vi "load engine runtime.vi"(8 "error in":errorcluster, 10 "engine configuration in":T1, 11 "Target Runtime in":refnum<class "PL_Target Runtime.lvclass">) -> (0 "error out":errorcluster, 1 "Module Runtime Objects":refnum<class "TBM module execution interface.lvclass">[](array[class]), 2 "Engine Runtime Object":refnum<class "Engine Runtime Interface.lvclass">, 3 "Target Runtime out":refnum<class "PL_Target Runtime.lvclass">)   [LabVIEW 2013, in "PL_Target Runtime.lvclass"]
doc: "A helper function which takes a single engine configuration (1 engine configuration object and N module configuration objects) and loads the runtime objects associated with each configuration object."
uses:
  PL_Target Runtime.lvclass
  platypus configuration/engines cluster.ctl
  <vilib>/NI/Module Execution Interface/Engine Configuration/engine configuration.lvclass
  <vilib>/NI/Tag Bus Module Framework/module configuration/TBM module configuration.lvclass
  <vilib>/NI/Module Execution Interface/Engine Runtime/Engine Runtime Interface.lvclass
  <vilib>/NI/Tag Bus Module Framework/runtime/TBM module execution interface.lvclass
  platypus configuration/PLConfigurationSerializer.lvlib
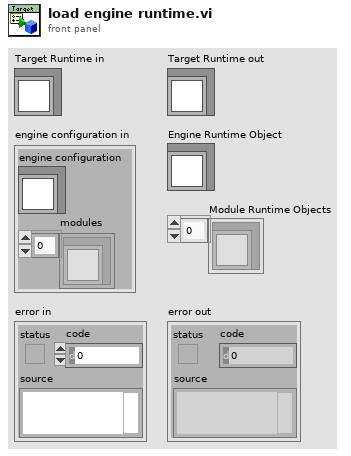
[diagram p1: front panel]
types:
  T1 = typedef "PLConfigurationSerializer.lvlib/engines cluster.ctl" = cluster{"engine configuration":refnum<class "engine configuration.lvclass">, "modules":refnum<class "TBM module configuration.lvclass">[]}
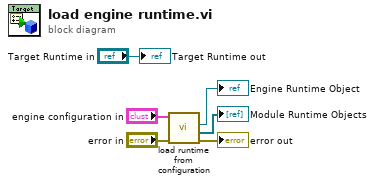
[diagram p0: block diagram]
diagram:
  n1 = call "load runtime from configuration.vi"("error in"="error in", "engine configuration in"="engine configuration in") -> ("error out"=→"error out":errorcluster, "Component Runtime Objects"=→"Module Runtime Objects":refnum<class "TBM module execution interface.lvclass">[], "Engine Runtime Object"=→"Engine Runtime Object":refnum<class "Engine Runtime Interface.lvclass">)  [unwired: 6 in, 1 out]
  "Target Runtime out" <- "Target Runtime in"
